vi "Wiener_HV_PowerSupplyWithLabVIEW.vi"() -> ()   [LabVIEW 2018]
panel:
  out "Numeric":i32
  in  "Tab Control":T1(tab)
  in  "IP":string="192.168.0.250"
  in  "stop":bool
  out "S1_Current":dbl[](array[numeric])
  out "S1_Voltage":dbl[](array[numeric])
  out "S2_Voltage":dbl[](array[numeric])
  out "S2_Current":dbl[](array[numeric])
  out "Start Time_L1":string
  out "S1_6-12 Channels Voltage":cluster{timestamp[], dbl[]}[](graph)
  out "S1_1-6 Channels Voltage":cluster{timestamp[], dbl[]}[](graph)
  out "S1_13-16 Channels Voltage":cluster{timestamp[], dbl[]}[](graph)
  in  "Clear_L1":bool
  out "Start Time_L2":string
  out "S1_13-16 Channels Current":cluster{timestamp[], dbl[]}[](graph)
  out "S1_1-6 Channels Current":cluster{timestamp[], dbl[]}[](graph)
  out "S1_6-12 Channels Current":cluster{timestamp[], dbl[]}[](graph)
  in  "Clear_L2":bool
  out "Start Time_L3":string
  out "S2_13-16 Channels Voltage":cluster{timestamp[], dbl[]}[](graph)
  out "S2_6-12 Channels Voltage":cluster{timestamp[], dbl[]}[](graph)
  out "S2_1-6 Channels Voltage":cluster{timestamp[], dbl[]}[](graph)
  in  "Clear_L3":bool
  out "Start Time_L4":string
  out "S2_1-6 Channels Current":cluster{timestamp[], dbl[]}[](graph)
  out "S2_6-12 Channels Current":cluster{timestamp[], dbl[]}[](graph)
  out "S2_13-16 Channels Current":cluster{timestamp[], dbl[]}[](graph)
  in  "Clear_L4":bool
  out "S1_V13":dbl format="%.2f"
  out "S1_V12":dbl format="%.2f"
  out "S1_V15":dbl format="%.2f"
  out "S1_V14":dbl format="%.2f"
  out "S1_I13":dbl format="%.2f"
  out "S1_I12":dbl format="%.2f"
  out "S1_I15":dbl format="%.2f"
  out "S1_I14":dbl format="%.2f"
  out "S1_I9":dbl format="%.2f"
  out "S1_I8":dbl format="%.2f"
  out "S1_I7":dbl format="%.2f"
  out "S1_I6":dbl format="%.2f"
  out "S1_V11":dbl format="%.2f"
  out "S1_V10":dbl format="%.2f"
  out "S1_V9":dbl format="%.2f"
  out "S1_V8":dbl format="%.2f"
  out "S1_V7":dbl format="%.2f"
  out "S1_V6":dbl format="%.2f"
  out "S1_I5":dbl format="%.2f"
  out "S1_I4":dbl format="%.2f"
  out "S1_I3":dbl format="%.2f"
  out "S1_I2":dbl format="%.2f"
  out "S1_I1":dbl format="%.2f"
  out "S1_V0":dbl format="%.2f"
  out "S1_V1":dbl format="%.2f"
  out "S1_V2":dbl format="%.2f"
  out "S1_V3":dbl format="%.2f"
  out "S1_V5":dbl format="%.2f"
  out "S1_V4":dbl format="%.2f"
  out "S1_I0":dbl format="%.2f"
  out "S1_I11":dbl format="%.2f"
  out "S1_I10":dbl format="%.2f"
  out "S2_V6":dbl format="%.2f"
  out "S2_V7":dbl format="%.2f"
  out "S2_V8":dbl format="%.2f"
  out "S2_V9":dbl format="%.2f"
  out "S2_V10":dbl format="%.2f"
  out "S2_V11":dbl format="%.2f"
  out "S2_I0":dbl format="%.2f"
  out "S2_I1":dbl format="%.2f"
  out "S2_I2":dbl format="%.2f"
  out "S2_I3":dbl format="%.2f"
  out "S2_I4":dbl format="%.2f"
  out "S2_I5":dbl format="%.2f"
  out "S2_I6":dbl format="%.2f"
  out "S2_I7":dbl format="%.2f"
  out "S2_I8":dbl format="%.2f"
  out "S2_I9":dbl format="%.2f"
  out "S2_I10":dbl format="%.2f"
  out "S2_I11":dbl format="%.2f"
  out "S2_I14":dbl format="%.2f"
  out "S2_I15":dbl format="%.2f"
  out "S2_I12":dbl format="%.2f"
  out "S2_I13":dbl format="%.2f"
  out "S2_V14":dbl format="%.2f"
  out "S2_V15":dbl format="%.2f"
  out "S2_V12":dbl format="%.2f"
  out "S2_V13":dbl format="%.2f"
  out "S2_V0":dbl format="%.2f"
  out "S2_V1":dbl format="%.2f"
  out "S2_V2":dbl format="%.2f"
  out "S2_V3":dbl format="%.2f"
  out "S2_V4":dbl format="%.2f"
  out "S2_V5":dbl format="%.2f"
  # "uA"
  # "V"
  # "uA"
  # "V"
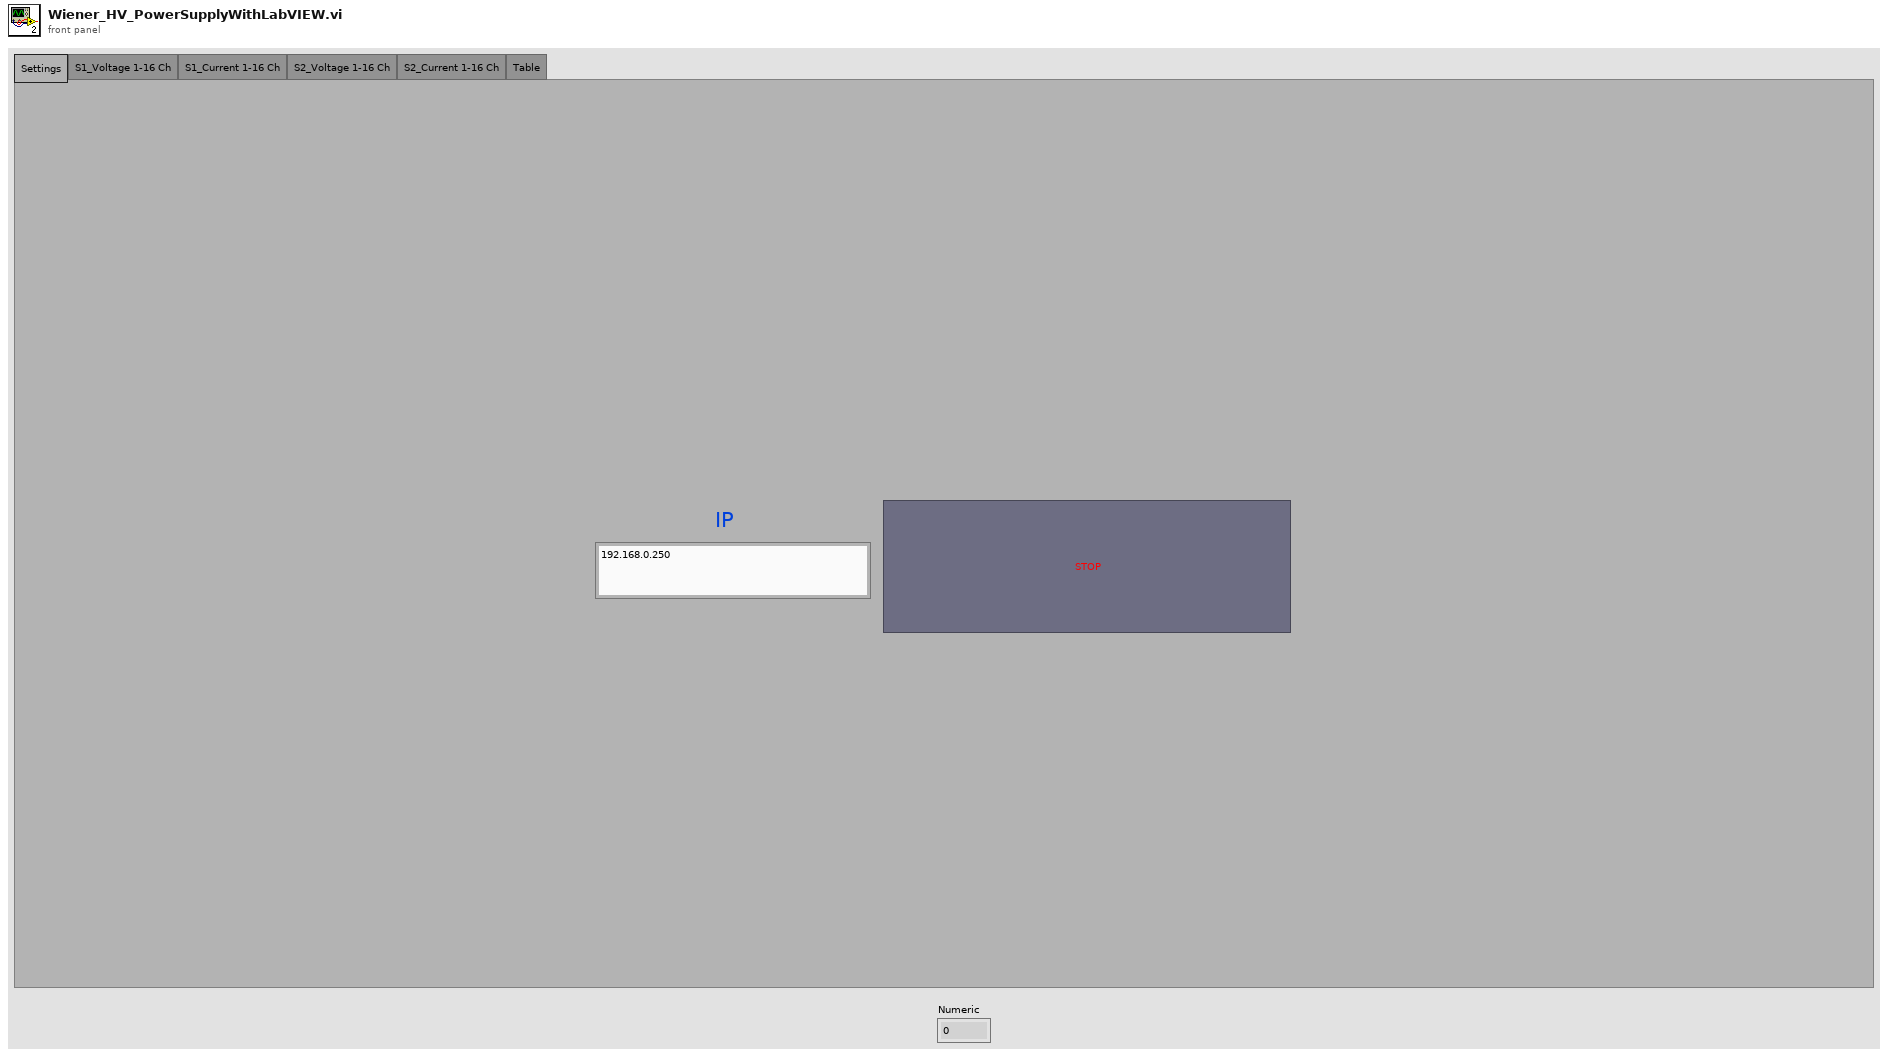
[diagram p1: front panel]
types:
  T1 = enum32{"Settings", "S1_Voltage 1-16 Ch", "S1_Current 1-16 Ch", "S2_Voltage 1-16 Ch", "S2_Current 1-16 Ch", "Table"}
  T2 = typedef "LVDateTimeRec.ctl" = cluster{"fractional second":dbl, "second":i32, "minute":i32, "hour":i32, "day of month":i32, "month":i32, "year":i32, "day of week":i32, "day of year":i32, "DST":i32}
  T3 = cluster{dbl, i32, i32, i32, "day of month":i32, "month":i32, "year":i32, "day of week":i32, "day of year":i32, "DST":i32}
  T4 = cluster{"fractional second":dbl, i32, i32, i32, "day of month":i32, "month":i32, "year":i32, "day of week":i32, "day of year":i32, "DST":i32}
  T5 = cluster{"appended array":timestamp[], "Ch 11":dbl[]}[]
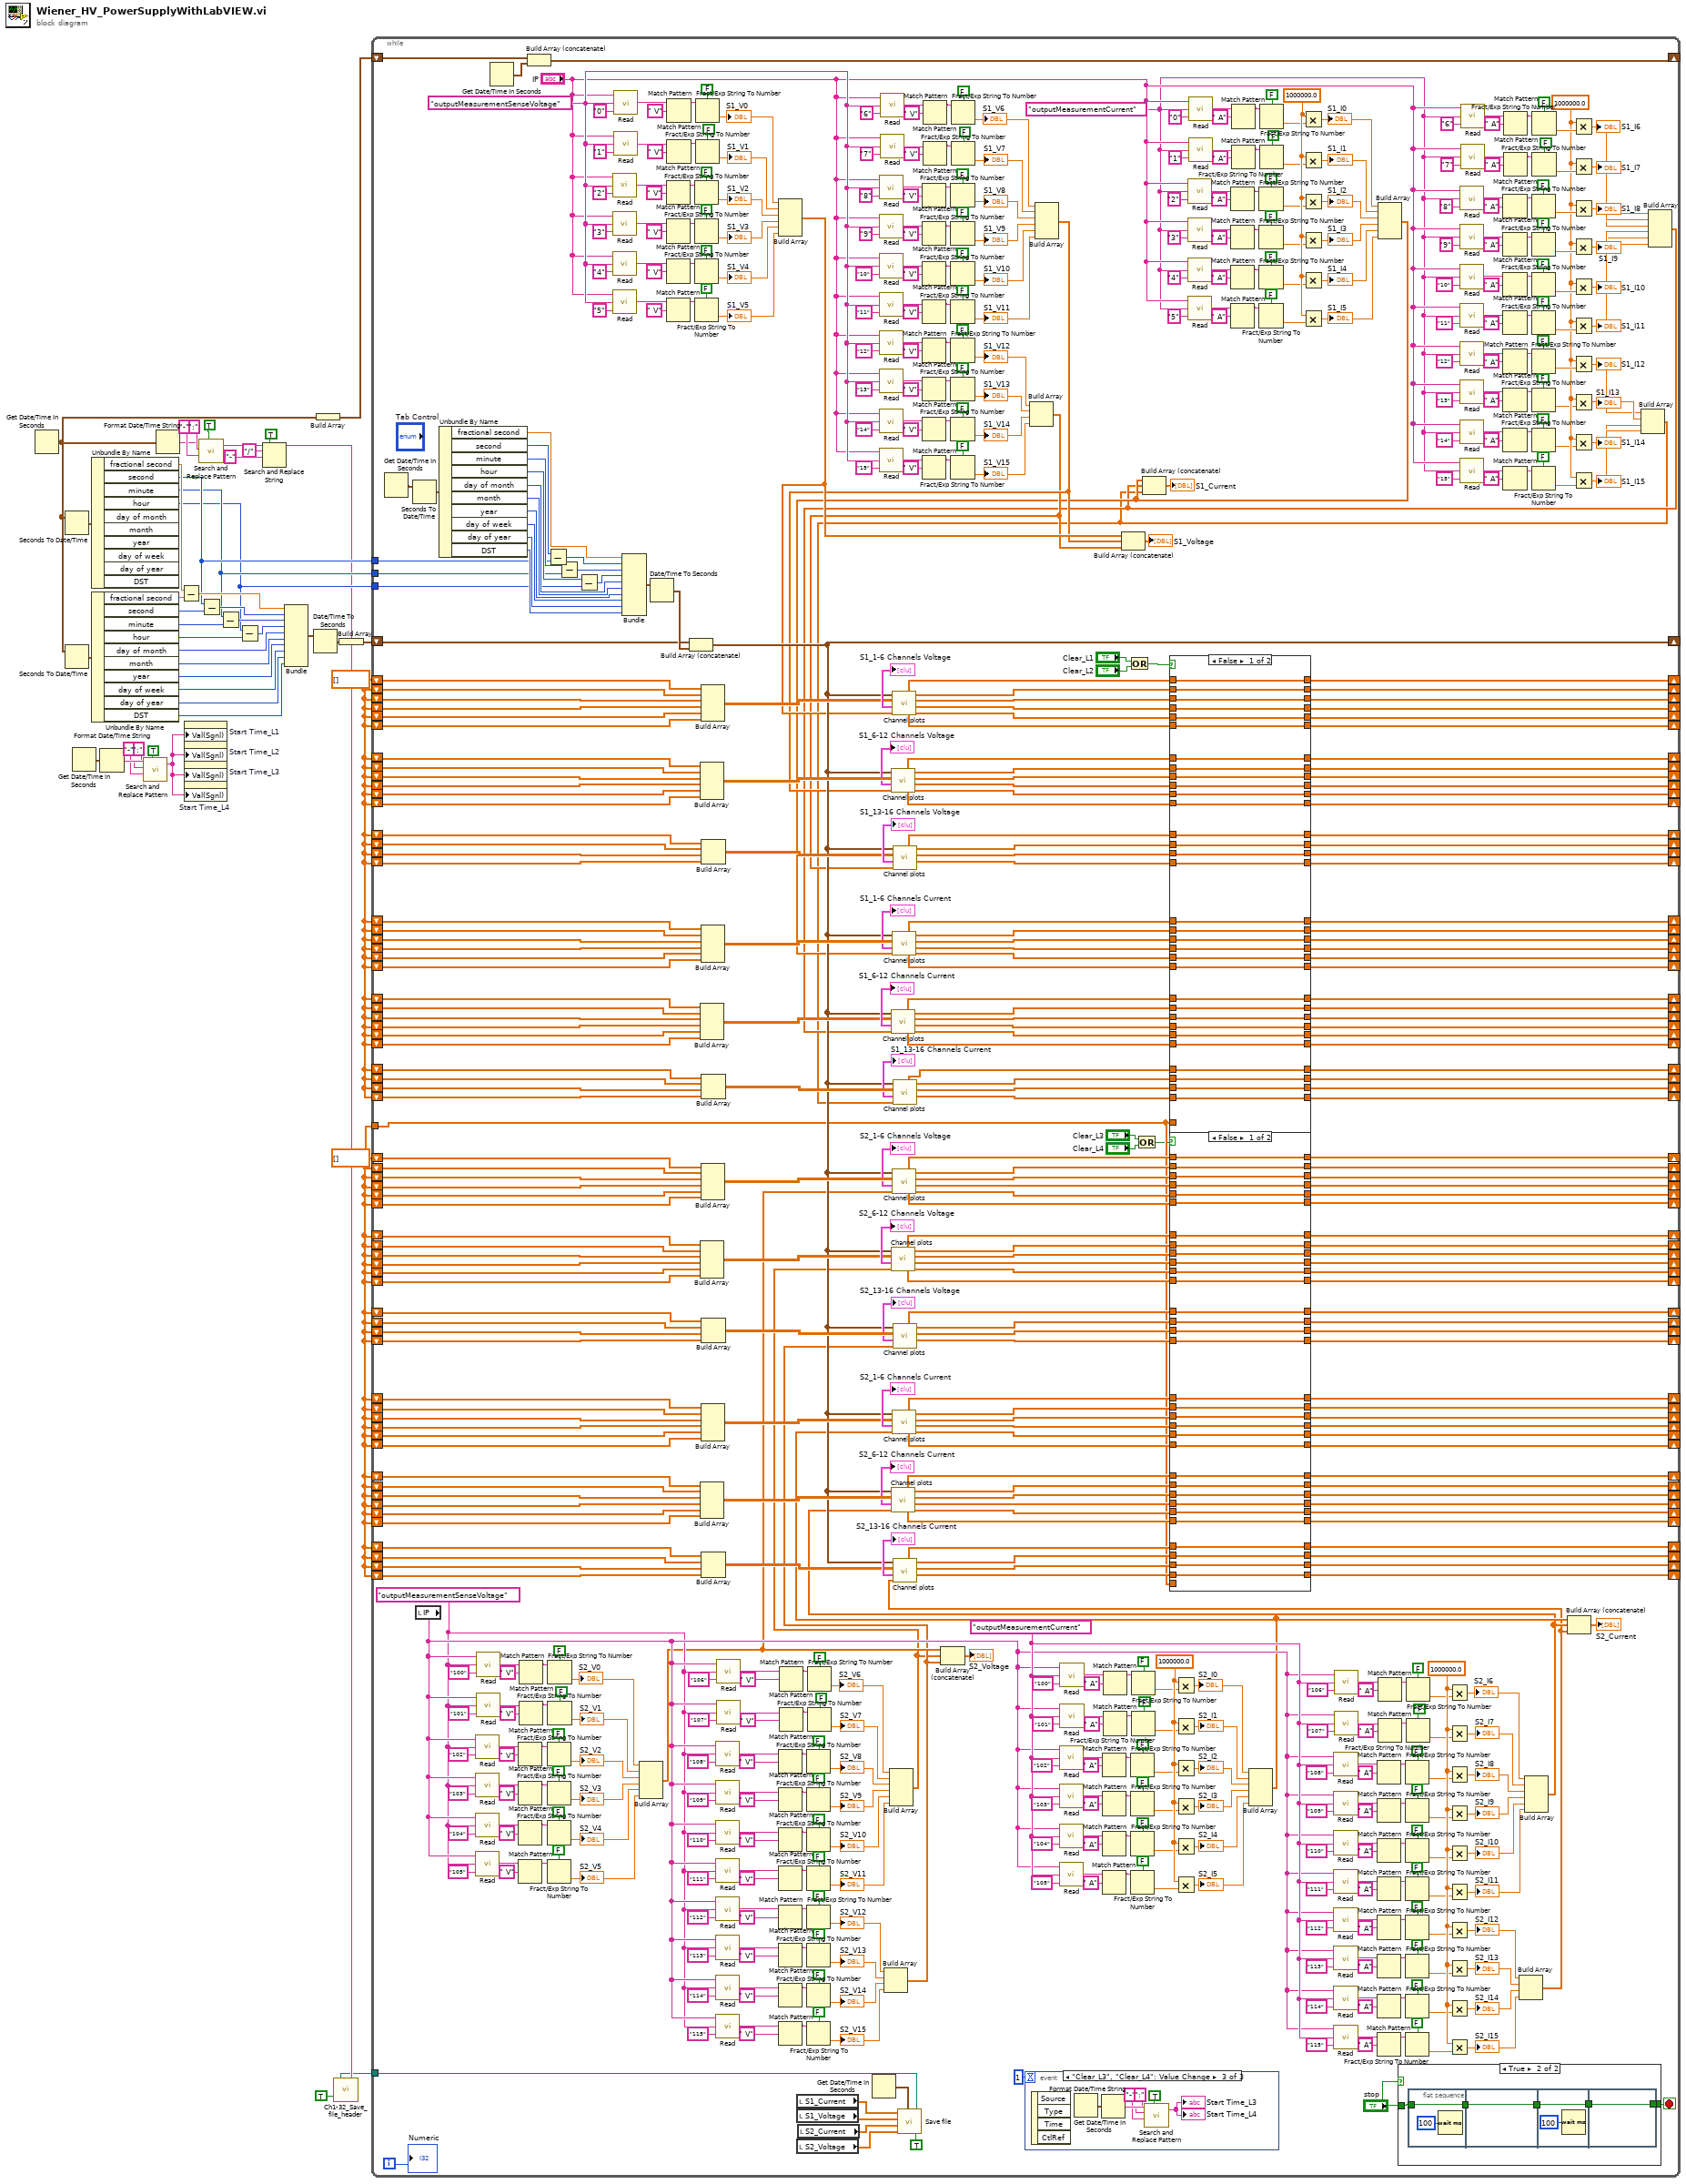
[diagram p0: block diagram]
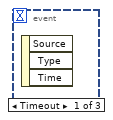
[diagram p3: hidden frame]
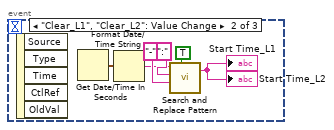
[diagram p4: hidden frame]
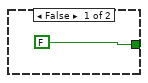
[diagram p6: hidden frame]
diagram:
  w8 = dbl[] [] ("out Ch 1")
  w15 = dbl[] [] ("out Ch 1")
  n1 = Get Date/Time In Seconds() -> (seconds since 1Jan1904=w18:timestamp)
  n2 = Seconds To Date/Time(time stamp (now)=w18) -> (date time rec=w26:T2)  [unwired: 1 in]
  n3 = Seconds To Date/Time(time stamp (now)=w18) -> (date time rec=w44:T2)  [unwired: 1 in]
  n4 = Get Date/Time In Seconds() -> (seconds since 1Jan1904=w6:timestamp)
  n5 = Unbundle By Name(w26) -> ("fractional second"=w29:dbl, "second"=w21:i32, "minute"=w20:i32, "hour"=w19:i32)  [unwired: 6 out]
  n6 = Unbundle By Name(w44) -> ("fractional second"=w43:dbl, "second"=w42:i32, "minute"=w41:i32, "hour"=w40:i32, "day of month"=w28:i32, "month"=w27:i32, "year"=w35:i32, "day of week"=w34:i32, "day of year"=w33:i32, "DST"=w32:i32)
  n7 = Format Date/Time String(seconds (now)=w6) -> (date/time string=w5:string)  [unwired: 2 in]
  n8 = call <vilib>:"Search and Replace Pattern.vi"("string"=w5, "regular expression (\"\")"=":" ("regular expression (\"\")"), "replace string (\"\")"="-" ("replace string (\"\")"), "replace all? (F)"=TRUE) -> ("result string"=w2:string)  [unwired: 1 in, 1 out]
  n9 = Format Date/Time String(seconds (now)=w18) -> (date/time string=w22:string)  [unwired: 2 in]
  n10 = Subtract(x=w29, y=w43) -> (x-y=w39:dbl)
  n11 = property on="Start Time_L1" class="Str"("Val(Sgnl)"=w2) -> ()  [unwired: 2 in, 2 out]
  n12 = property on="Start Time_L2" class="Str"("Val(Sgnl)"=w2) -> ()  [unwired: 2 in, 2 out]
  n13 = property on="Start Time_L3" class="Str"("Val(Sgnl)"=w2) -> ()  [unwired: 2 in, 2 out]
  n14 = property on="Start Time_L4" class="Str"("Val(Sgnl)"=w2) -> ()  [unwired: 2 in, 2 out]
  n15 = call <vilib>:"Search and Replace Pattern.vi"("string"=w22, "regular expression (\"\")"=":" ("regular expression (\"\")"), "replace string (\"\")"="-" ("replace string (\"\")"), "replace all? (F)"=TRUE) -> ("result string"=w13:string)  [unwired: 1 in, 1 out]
  n16 = Subtract(x=w21, y=w42) -> (x-y=w38:i32)
  n17 = Subtract(x=w20, y=w41) -> (x-y=w37:i32)
  n18 = Subtract(x=w19, y=w40) -> (x-y=w36:i32)
  n19 = Search and Replace String(replace all?=TRUE ("replace all? (F)"), input string=w13, search string="/", replace string="-" ("replace string (\"\")")) -> (result string=w9:string)  [unwired: 4 in, 3 out]
  n20 = Bundle(w39, w38, w37, w36, "day of month"=w28, "month"=w27, "year"=w35, "day of week"=w34, "day of year"=w33, "DST"=w32) -> (w30:T3)  [unwired: 1 in]
  n21 = Date/Time To Seconds(2:w30) -> (0:w31:timestamp)  [unwired: 1 in]
  n22 = Build Array(w18) -> (w17:timestamp[])
  n23 = call "Ch1-32_Save_file_header.vi"("File name"=w9, "Save"=TRUE) -> ("Output Path"=w1:path)
  n24 = Build Array(w31) -> (w16:timestamp[])
  n25 = while {
    tunnel: w21 -> [w725]
    tunnel: w20 -> [w724]
    tunnel: w19 -> [w723]
    shift-right: [w720] -> _
    shift-left: w17 -> [w722]
    shift-right: [w460] -> _
    shift-left: w16 -> [w718]
    shift-right: [w262] -> _
    shift-left: w15 -> [w715]
    shift-right: [w261] -> _
    shift-left: w15 -> [w714]
    shift-right: [w258] -> _
    shift-left: w15 -> [w713]
    shift-right: [w256] -> _
    shift-left: w15 -> [w712]
    shift-right: [w254] -> _
    shift-left: w15 -> [w711]
    shift-right: [w253] -> _
    shift-left: w15 -> [w710]
    shift-right: [w250] -> _
    shift-left: w15 -> [w642]
    shift-right: [w248] -> _
    shift-left: w15 -> [w643]
    shift-right: [w246] -> _
    shift-left: w15 -> [w644]
    shift-right: [w244] -> _
    shift-left: w15 -> [w645]
    shift-right: [w242] -> _
    shift-left: w15 -> [w646]
    shift-right: [w240] -> _
    shift-left: w15 -> [w647]
    shift-right: [w230] -> _
    shift-left: w15 -> [w566]
    shift-right: [w228] -> _
    shift-left: w15 -> [w567]
    shift-right: [w226] -> _
    shift-left: w15 -> [w568]
    shift-right: [w224] -> _
    shift-left: w15 -> [w569]
    shift-right: [w222] -> _
    shift-left: w15 -> [w570]
    shift-right: [w220] -> _
    shift-left: w15 -> [w571]
    shift-right: [w218] -> _
    shift-left: w15 -> [w577]
    shift-right: [w216] -> _
    shift-left: w15 -> [w576]
    shift-right: [w214] -> _
    shift-left: w15 -> [w575]
    shift-right: [w212] -> _
    shift-left: w15 -> [w574]
    shift-right: [w210] -> _
    shift-left: w15 -> [w573]
    shift-right: [w208] -> _
    shift-left: w15 -> [w572]
    shift-right: [w238] -> _
    shift-left: w15 -> [w561]
    shift-right: [w236] -> _
    shift-left: w15 -> [w560]
    shift-right: [w234] -> _
    shift-left: w15 -> [w559]
    shift-right: [w232] -> _
    shift-left: w15 -> [w558]
    shift-right: [w206] -> _
    shift-left: w15 -> [w507]
    shift-right: [w204] -> _
    shift-left: w15 -> [w508]
    shift-right: [w202] -> _
    shift-left: w15 -> [w509]
    shift-right: [w200] -> _
    shift-left: w15 -> [w510]
    shift-right: [w194] -> _
    shift-left: w8 -> [w463]
    shift-right: [w192] -> _
    shift-left: w8 -> [w464]
    shift-right: [w190] -> _
    shift-left: w8 -> [w465]
    shift-right: [w188] -> _
    shift-left: w8 -> [w466]
    shift-right: [w186] -> _
    shift-left: w8 -> [w467]
    shift-right: [w184] -> _
    shift-left: w8 -> [w468]
    shift-right: [w182] -> _
    shift-left: w8 -> [w474]
    shift-right: [w180] -> _
    shift-left: w8 -> [w473]
    shift-right: [w178] -> _
    shift-left: w8 -> [w472]
    shift-right: [w176] -> _
    shift-left: w8 -> [w471]
    shift-right: [w174] -> _
    shift-left: w8 -> [w470]
    shift-right: [w172] -> _
    shift-left: w8 -> [w469]
    shift-right: [w162] -> _
    shift-left: w8 -> [w490]
    shift-right: [w160] -> _
    shift-left: w8 -> [w489]
    shift-right: [w158] -> _
    shift-left: w8 -> [w488]
    shift-right: [w156] -> _
    shift-left: w8 -> [w487]
    shift-right: [w154] -> _
    shift-left: w8 -> [w486]
    shift-right: [w152] -> _
    shift-left: w8 -> [w485]
    shift-right: [w150] -> _
    shift-left: w8 -> [w479]
    shift-right: [w148] -> _
    shift-left: w8 -> [w480]
    shift-right: [w146] -> _
    shift-left: w8 -> [w481]
    shift-right: [w144] -> _
    shift-left: w8 -> [w482]
    shift-right: [w142] -> _
    shift-left: w8 -> [w483]
    shift-right: [w140] -> _
    shift-left: w8 -> [w484]
    shift-right: [w170] -> _
    shift-left: w8 -> [w495]
    shift-right: [w168] -> _
    shift-left: w8 -> [w496]
    shift-right: [w166] -> _
    shift-left: w8 -> [w497]
    shift-right: [w164] -> _
    shift-left: w8 -> [w498]
    shift-right: [w138] -> _
    shift-left: w8 -> [w502]
    shift-right: [w136] -> _
    shift-left: w8 -> [w501]
    shift-right: [w134] -> _
    shift-left: w8 -> [w500]
    shift-right: [w132] -> _
    shift-left: w8 -> [w499]
    tunnel: w8 -> [w130]
    tunnel: w1 -> [w47]
    i -> [w45]
    stop <- w264 stop-if-true
    w73 = 1000000.0 ("x")
    w86 = 1000000.0 ("x")
    w93 = 1000000.0 ("x")
    w126 = 1000000.0 ("x")
    w281 = "outputMeasurementSenseVoltage" ("R_Call_Function_Voltage")
    w283 = "outputMeasurementCurrent" ("R_Call_Function_Voltage")
    w511 = "outputMeasurementCurrent" ("R_Call_Function_Voltage")
    w537 = "outputMeasurementSenseVoltage" ("R_Call_Function_Voltage")
    n26 = Get Date/Time In Seconds() -> (seconds since 1Jan1904=w741:timestamp)
    n27 = Seconds To Date/Time(time stamp (now)=w741) -> (date time rec=w740:T2)  [unwired: 1 in]
    n28 = local read "IP"() -> (w282:string)
    n29 = Unbundle By Name(w740) -> ("fractional second"=w726:dbl, "second"=w736:i32, "minute"=w735:i32, "hour"=w734:i32, "day of month"=w733:i32, "month"=w732:i32, "year"=w731:i32, "day of week"=w730:i32, "day of year"=w729:i32, "DST"=w728:i32)
    n30 = call "Read.vi"("R_Channel"="102", "R_Call_Function"=w281, "IP"=w282) -> ("R_Return"=w447:string)
    n31 = call "Read.vi"("R_Channel"="103", "R_Call_Function"=w281, "IP"=w282) -> ("R_Return"=w445:string)
    n32 = call "Read.vi"("R_Channel"="104", "R_Call_Function"=w281, "IP"=w282) -> ("R_Return"=w435:string)
    n33 = call "Read.vi"("R_Channel"="105", "R_Call_Function"=w281, "IP"=w282) -> ("R_Return"=w436:string)
    n34 = call "Read.vi"("R_Channel"="100", "R_Call_Function"=w281, "IP"=w282) -> ("R_Return"=w456:string)
    n35 = call "Read.vi"("R_Channel"="101", "R_Call_Function"=w281, "IP"=w282) -> ("R_Return"=w446:string)
    n36 = Get Date/Time In Seconds() -> (seconds since 1Jan1904=w721:timestamp)
    n37 = Match Pattern(string=w447, regular expression=" V") -> (before substring=w448:string)  [unwired: 1 in, 3 out]
    n38 = Match Pattern(string=w445, regular expression=" V") -> (before substring=w444:string)  [unwired: 1 in, 3 out]
    n39 = Match Pattern(string=w435, regular expression=" V") -> (before substring=w434:string)  [unwired: 1 in, 3 out]
    n40 = Match Pattern(string=w436, regular expression=" V") -> (before substring=w437:string)  [unwired: 1 in, 3 out]
    n41 = Match Pattern(string=w456, regular expression=" V") -> (before substring=w457:string)  [unwired: 1 in, 3 out]
    n42 = Match Pattern(string=w446, regular expression=" V") -> (before substring=w455:string)  [unwired: 1 in, 3 out]
    n43 = Build Array (concatenate)(w722, w721) -> (w720:timestamp[])
    n44 = Subtract(x=w736, y=w725) -> (x-y=w737:i32)
    n45 = Fract/Exp String To Number(use system decimal point (T)=FALSE, string=w448) -> (number=w428:dbl)  [unwired: 2 in, 1 out]
    "S2_V2" <- w428
    n46 = Fract/Exp String To Number(use system decimal point (T)=FALSE, string=w444) -> (number=w427:dbl)  [unwired: 2 in, 1 out]
    "S2_V3" <- w427
    n47 = Fract/Exp String To Number(use system decimal point (T)=FALSE, string=w434) -> (number=w426:dbl)  [unwired: 2 in, 1 out]
    "S2_V4" <- w426
    n48 = Fract/Exp String To Number(use system decimal point (T)=FALSE, string=w437) -> (number=w425:dbl)  [unwired: 2 in, 1 out]
    "S2_V5" <- w425
    n49 = Fract/Exp String To Number(use system decimal point (T)=FALSE, string=w457) -> (number=w430:dbl)  [unwired: 2 in, 1 out]
    "S2_V0" <- w430
    n50 = Fract/Exp String To Number(use system decimal point (T)=FALSE, string=w455) -> (number=w429:dbl)  [unwired: 2 in, 1 out]
    "S2_V1" <- w429
    n51 = Subtract(x=w735, y=w724) -> (x-y=w738:i32)
    n52 = Subtract(x=w734, y=w723) -> (x-y=w739:i32)
    n53 = call "Read.vi"("R_Channel"="2", "R_Call_Function"=w537, "IP"="IP") -> ("R_Return"=w701:string)
    n54 = call "Read.vi"("R_Channel"="3", "R_Call_Function"=w537, "IP"="IP") -> ("R_Return"=w699:string)
    n55 = call "Read.vi"("R_Channel"="4", "R_Call_Function"=w537, "IP"="IP") -> ("R_Return"=w689:string)
    n56 = call "Read.vi"("R_Channel"="5", "R_Call_Function"=w537, "IP"="IP") -> ("R_Return"=w690:string)
    n57 = call "Read.vi"("R_Channel"="0", "R_Call_Function"=w537, "IP"="IP") -> ("R_Return"=w742:string)
    n58 = call "Read.vi"("R_Channel"="1", "R_Call_Function"=w537, "IP"="IP") -> ("R_Return"=w700:string)
    n59 = Bundle("fractional second"=w726, w737, w738, w739, "day of month"=w733, "month"=w732, "year"=w731, "day of week"=w730, "day of year"=w729, "DST"=w728) -> (w727:T4)  [unwired: 1 in]
    n60 = Build Array(w430, w429, w428, w427, w426, w425) -> (w274:dbl[])
    n61 = Date/Time To Seconds(2:w727) -> (0:w719:timestamp)  [unwired: 1 in]
    n62 = Match Pattern(string=w701, regular expression=" V") -> (before substring=w702:string)  [unwired: 1 in, 3 out]
    n63 = Match Pattern(string=w699, regular expression=" V") -> (before substring=w698:string)  [unwired: 1 in, 3 out]
    n64 = Match Pattern(string=w689, regular expression=" V") -> (before substring=w688:string)  [unwired: 1 in, 3 out]
    n65 = Match Pattern(string=w690, regular expression=" V") -> (before substring=w691:string)  [unwired: 1 in, 3 out]
    n66 = Match Pattern(string=w742, regular expression=" V") -> (before substring=w743:string)  [unwired: 1 in, 3 out]
    n67 = Match Pattern(string=w700, regular expression=" V") -> (before substring=w709:string)  [unwired: 1 in, 3 out]
    n68 = Build Array (concatenate)(w718, w719) -> (w460:timestamp[])
    n69 = Fract/Exp String To Number(use system decimal point (T)=FALSE, string=w702) -> (number=w122:dbl)  [unwired: 2 in, 1 out]
    "S1_V2" <- w122
    n70 = Fract/Exp String To Number(use system decimal point (T)=FALSE, string=w698) -> (number=w123:dbl)  [unwired: 2 in, 1 out]
    "S1_V3" <- w123
    n71 = Fract/Exp String To Number(use system decimal point (T)=FALSE, string=w688) -> (number=w125:dbl)  [unwired: 2 in, 1 out]
    "S1_V4" <- w125
    n72 = Fract/Exp String To Number(use system decimal point (T)=FALSE, string=w691) -> (number=w124:dbl)  [unwired: 2 in, 1 out]
    "S1_V5" <- w124
    n73 = Fract/Exp String To Number(use system decimal point (T)=FALSE, string=w743) -> (number=w120:dbl)  [unwired: 2 in, 1 out]
    "S1_V0" <- w120
    n74 = Fract/Exp String To Number(use system decimal point (T)=FALSE, string=w709) -> (number=w121:dbl)  [unwired: 2 in, 1 out]
    "S1_V1" <- w121
    n75 = Build Array(w642, w643, w644, w645, w646, w647) -> (w641:dbl[][])
    n76 = Build Array(w577, w576, w575, w574, w573, w572) -> (w578:dbl[][])
    n77 = Build Array(w474, w473, w472, w471, w470, w469) -> (w475:dbl[][])
    n78 = Build Array(w479, w480, w481, w482, w483, w484) -> (w478:dbl[][])
    n79 = Build Array(w715, w714, w713, w712, w711, w710) -> (w716:dbl[][])
    n80 = Build Array(w566, w567, w568, w569, w570, w571) -> (w565:dbl[][])
    n81 = Build Array(w463, w464, w465, w466, w467, w468) -> (w462:dbl[][])
    n82 = Build Array(w490, w489, w488, w487, w486, w485) -> (w491:dbl[][])
    n83 = Build Array(w561, w560, w559, w558) -> (w562:dbl[][])
    n84 = Build Array(w507, w508, w509, w510) -> (w506:dbl[][])
    n85 = Build Array(w495, w496, w497, w498) -> (w494:dbl[][])
    n86 = Build Array(w502, w501, w500, w499) -> (w503:dbl[][])
    n87 = call "Read.vi"("R_Channel"="108", "R_Call_Function"=w281, "IP"=w282) -> ("R_Return"=w400:string)
    n88 = call "Read.vi"("R_Channel"="109", "R_Call_Function"=w281, "IP"=w282) -> ("R_Return"=w402:string)
    n89 = call "Read.vi"("R_Channel"="110", "R_Call_Function"=w281, "IP"=w282) -> ("R_Return"=w412:string)
    n90 = call "Read.vi"("R_Channel"="111", "R_Call_Function"=w281, "IP"=w282) -> ("R_Return"=w411:string)
    n91 = call "Read.vi"("R_Channel"="112", "R_Call_Function"=w281, "IP"=w282) -> ("R_Return"=w323:string)
    n92 = call "Read.vi"("R_Channel"="113", "R_Call_Function"=w281, "IP"=w282) -> ("R_Return"=w322:string)
    n93 = call "Read.vi"("R_Channel"="114", "R_Call_Function"=w281, "IP"=w282) -> ("R_Return"=w312:string)
    n94 = call "Read.vi"("R_Channel"="115", "R_Call_Function"=w281, "IP"=w282) -> ("R_Return"=w313:string)
    n95 = call "Read.vi"("R_Channel"="106", "R_Call_Function"=w281, "IP"=w282) -> ("R_Return"=w391:string)
    n96 = call "Read.vi"("R_Channel"="107", "R_Call_Function"=w281, "IP"=w282) -> ("R_Return"=w401:string)
    n97 = Build Array(w120, w121, w122, w123, w125, w124) -> (w280:dbl[])
    n98 = Match Pattern(string=w400, regular expression=" V") -> (before substring=w399:string)  [unwired: 1 in, 3 out]
    n99 = Match Pattern(string=w402, regular expression=" V") -> (before substring=w403:string)  [unwired: 1 in, 3 out]
    n100 = Match Pattern(string=w412, regular expression=" V") -> (before substring=w413:string)  [unwired: 1 in, 3 out]
    n101 = Match Pattern(string=w411, regular expression=" V") -> (before substring=w410:string)  [unwired: 1 in, 3 out]
    n102 = Match Pattern(string=w323, regular expression=" V") -> (before substring=w324:string)  [unwired: 1 in, 3 out]
    n103 = Match Pattern(string=w322, regular expression=" V") -> (before substring=w321:string)  [unwired: 1 in, 3 out]
    n104 = Match Pattern(string=w312, regular expression=" V") -> (before substring=w311:string)  [unwired: 1 in, 3 out]
    n105 = Match Pattern(string=w313, regular expression=" V") -> (before substring=w314:string)  [unwired: 1 in, 3 out]
    n106 = Match Pattern(string=w391, regular expression=" V") -> (before substring=w390:string)  [unwired: 1 in, 3 out]
    n107 = Match Pattern(string=w401, regular expression=" V") -> (before substring=w392:string)  [unwired: 1 in, 3 out]
    n108 = local read "S1_Current"() -> (w49:dbl[])
    n109 = local read "S1_Voltage"() -> (w50:dbl[])
    n110 = local read "S2_Voltage"() -> (w52:dbl[])
    n111 = local read "S2_Current"() -> (w51:dbl[])
    n112 = Fract/Exp String To Number(use system decimal point (T)=FALSE, string=w399) -> (number=w419:dbl)  [unwired: 2 in, 1 out]
    "S2_V8" <- w419
    n113 = Fract/Exp String To Number(use system decimal point (T)=FALSE, string=w403) -> (number=w420:dbl)  [unwired: 2 in, 1 out]
    "S2_V9" <- w420
    n114 = Fract/Exp String To Number(use system decimal point (T)=FALSE, string=w413) -> (number=w421:dbl)  [unwired: 2 in, 1 out]
    "S2_V10" <- w421
    n115 = Fract/Exp String To Number(use system decimal point (T)=FALSE, string=w410) -> (number=w422:dbl)  [unwired: 2 in, 1 out]
    "S2_V11" <- w422
    n116 = Fract/Exp String To Number(use system decimal point (T)=FALSE, string=w324) -> (number=w307:dbl)  [unwired: 2 in, 1 out]
    "S2_V12" <- w307
    n117 = Fract/Exp String To Number(use system decimal point (T)=FALSE, string=w321) -> (number=w306:dbl)  [unwired: 2 in, 1 out]
    "S2_V13" <- w306
    n118 = Fract/Exp String To Number(use system decimal point (T)=FALSE, string=w311) -> (number=w305:dbl)  [unwired: 2 in, 1 out]
    "S2_V14" <- w305
    n119 = Fract/Exp String To Number(use system decimal point (T)=FALSE, string=w314) -> (number=w304:dbl)  [unwired: 2 in, 1 out]
    "S2_V15" <- w304
    n120 = Fract/Exp String To Number(use system decimal point (T)=FALSE, string=w390) -> (number=w417:dbl)  [unwired: 2 in, 1 out]
    "S2_V6" <- w417
    n121 = Fract/Exp String To Number(use system decimal point (T)=FALSE, string=w392) -> (number=w418:dbl)  [unwired: 2 in, 1 out]
    "S2_V7" <- w418
    n122 = Get Date/Time In Seconds() -> (seconds since 1Jan1904=w48:timestamp)
    n123 = call "Read.vi"("R_Channel"="8", "R_Call_Function"=w537, "IP"="IP") -> ("R_Return"=w660:string)
    n124 = call "Read.vi"("R_Channel"="9", "R_Call_Function"=w537, "IP"="IP") -> ("R_Return"=w662:string)
    n125 = call "Read.vi"("R_Channel"="10", "R_Call_Function"=w537, "IP"="IP") -> ("R_Return"=w672:string)
    n126 = call "Read.vi"("R_Channel"="11", "R_Call_Function"=w537, "IP"="IP") -> ("R_Return"=w671:string)
    n127 = call "Read.vi"("R_Channel"="12", "R_Call_Function"=w537, "IP"="IP") -> ("R_Return"=w553:string)
    n128 = call "Read.vi"("R_Channel"="13", "R_Call_Function"=w537, "IP"="IP") -> ("R_Return"=w552:string)
    n129 = call "Read.vi"("R_Channel"="14", "R_Call_Function"=w537, "IP"="IP") -> ("R_Return"=w542:string)
    n130 = call "Read.vi"("R_Channel"="15", "R_Call_Function"=w537, "IP"="IP") -> ("R_Return"=w543:string)
    n131 = call "Read.vi"("R_Channel"="6", "R_Call_Function"=w537, "IP"="IP") -> ("R_Return"=w651:string)
    n132 = call "Read.vi"("R_Channel"="7", "R_Call_Function"=w537, "IP"="IP") -> ("R_Return"=w661:string)
    n133 = Build Array(w307, w306, w305, w304) -> (w273:dbl[])
    n134 = Build Array(w417, w418, w419, w420, w421, w422) -> (w131:dbl[])
    n135 = call "Channel plots.vi"("Current time"=w460, "In Channels"=w475, "Input Channels"=w131) -> ("output graph"=→"S2_6-12 Channels Voltage":T5, "out Ch 1"=w183:dbl[], "out Ch 6"=w173:dbl[], "out Ch 2"=w181:dbl[], "out Ch 3"=w179:dbl[], "out Ch 4"=w177:dbl[], "out Ch 5"=w175:dbl[])
    n136 = call "Channel plots.vi"("Current time"=w460, "In Channels"=w716, "Input Channels"=w280) -> ("output graph"=→"S1_1-6 Channels Voltage":T5, "out Ch 1"=w263:dbl[], "out Ch 6"=w252:dbl[], "out Ch 2"=w260:dbl[], "out Ch 3"=w259:dbl[], "out Ch 4"=w257:dbl[], "out Ch 5"=w255:dbl[])
    n137 = call "Channel plots.vi"("Current time"=w460, "In Channels"=w462, "Input Channels"=w274) -> ("output graph"=→"S2_1-6 Channels Voltage":T5, "out Ch 1"=w195:dbl[], "out Ch 6"=w185:dbl[], "out Ch 2"=w193:dbl[], "out Ch 3"=w191:dbl[], "out Ch 4"=w189:dbl[], "out Ch 5"=w187:dbl[])
    n138 = call "Channel plots.vi"("Current time"=w460, "In Channels"=w494, "Input Channels"=w273) -> ("output graph"=→"S2_13-16 Channels Voltage":T5, "out Ch 1"=w171:dbl[], "out Ch 2"=w169:dbl[], "out Ch 3"=w167:dbl[], "out Ch 4"=w165:dbl[])  [unwired: 2 out]
    n139 = call "Save file.vi"("S1_Current"=w49, "S1_Voltage"=w50, "S2_Current"=w51, "S2_Voltage"=w52, "current time"=w48, "Save path"=w47, "Save"=TRUE) -> ()
    n140 = Match Pattern(string=w660, regular expression=" V") -> (before substring=w659:string)  [unwired: 1 in, 3 out]
    n141 = Match Pattern(string=w662, regular expression=" V") -> (before substring=w663:string)  [unwired: 1 in, 3 out]
    n142 = Match Pattern(string=w672, regular expression=" V") -> (before substring=w673:string)  [unwired: 1 in, 3 out]
    n143 = Match Pattern(string=w671, regular expression=" V") -> (before substring=w670:string)  [unwired: 1 in, 3 out]
    n144 = Match Pattern(string=w553, regular expression=" V") -> (before substring=w554:string)  [unwired: 1 in, 3 out]
    n145 = Match Pattern(string=w552, regular expression=" V") -> (before substring=w551:string)  [unwired: 1 in, 3 out]
    n146 = Match Pattern(string=w542, regular expression=" V") -> (before substring=w541:string)  [unwired: 1 in, 3 out]
    n147 = Match Pattern(string=w543, regular expression=" V") -> (before substring=w544:string)  [unwired: 1 in, 3 out]
    n148 = Match Pattern(string=w651, regular expression=" V") -> (before substring=w650:string)  [unwired: 1 in, 3 out]
    n149 = Match Pattern(string=w661, regular expression=" V") -> (before substring=w652:string)  [unwired: 1 in, 3 out]
    n150 = Build Array (concatenate)(w274, w131, w273) -> (→"S2_Voltage":dbl[])
    n151 = Fract/Exp String To Number(use system decimal point (T)=FALSE, string=w659) -> (number=w679:dbl)  [unwired: 2 in, 1 out]
    "S1_V8" <- w679
    n152 = Fract/Exp String To Number(use system decimal point (T)=FALSE, string=w663) -> (number=w680:dbl)  [unwired: 2 in, 1 out]
    "S1_V9" <- w680
    n153 = Fract/Exp String To Number(use system decimal point (T)=FALSE, string=w673) -> (number=w681:dbl)  [unwired: 2 in, 1 out]
    "S1_V10" <- w681
    n154 = Fract/Exp String To Number(use system decimal point (T)=FALSE, string=w670) -> (number=w682:dbl)  [unwired: 2 in, 1 out]
    "S1_V11" <- w682
    n155 = Fract/Exp String To Number(use system decimal point (T)=FALSE, string=w554) -> (number=w536:dbl)  [unwired: 2 in, 1 out]
    "S1_V12" <- w536
    n156 = Fract/Exp String To Number(use system decimal point (T)=FALSE, string=w551) -> (number=w535:dbl)  [unwired: 2 in, 1 out]
    "S1_V13" <- w535
    n157 = Fract/Exp String To Number(use system decimal point (T)=FALSE, string=w541) -> (number=w534:dbl)  [unwired: 2 in, 1 out]
    "S1_V14" <- w534
    n158 = Fract/Exp String To Number(use system decimal point (T)=FALSE, string=w544) -> (number=w533:dbl)  [unwired: 2 in, 1 out]
    "S1_V15" <- w533
    n159 = Fract/Exp String To Number(use system decimal point (T)=FALSE, string=w650) -> (number=w677:dbl)  [unwired: 2 in, 1 out]
    "S1_V6" <- w677
    n160 = Fract/Exp String To Number(use system decimal point (T)=FALSE, string=w652) -> (number=w678:dbl)  [unwired: 2 in, 1 out]
    "S1_V7" <- w678
    n161 = event shown="[2] \"Clear_L3\", \"Clear_L4\": Value Change" {
      selector: _ -> [_ _ _]
      dyn-events: _ -> [_ _ _]
      timeout: 1 -> [_ _ _]
      event Timeout {
        n162 = event-data() -> ()  [unwired: 1 in, 3 out]
      }
      event "Clear_L1", "Clear_L2": Value Change {
        n163 = event-data() -> ()  [unwired: 1 in, 5 out]
        n164 = Get Date/Time In Seconds() -> (seconds since 1Jan1904=w781:timestamp)
        n165 = Format Date/Time String(seconds (now)=w781) -> (date/time string=w782:string)  [unwired: 2 in]
        n166 = call <vilib>:"Search and Replace Pattern.vi"("string"=w782, "regular expression (\"\")"=":" ("regular expression (\"\")"), "replace string (\"\")"="-" ("replace string (\"\")"), "replace all? (F)"=TRUE) -> ("result string"=→"Start Time_L1" →"Start Time_L2":string)  [unwired: 1 in, 1 out]
      }
      event "Clear_L3", "Clear_L4": Value Change {
        n167 = event-data() -> ()  [unwired: 1 in, 4 out]
        n168 = Get Date/Time In Seconds() -> (seconds since 1Jan1904=w789:timestamp)
        n169 = Format Date/Time String(seconds (now)=w789) -> (date/time string=w790:string)  [unwired: 2 in]
        n170 = call <vilib>:"Search and Replace Pattern.vi"("string"=w790, "regular expression (\"\")"=":" ("regular expression (\"\")"), "replace string (\"\")"="-" ("replace string (\"\")"), "replace all? (F)"=TRUE) -> ("result string"=→"Start Time_L3" →"Start Time_L4":string)  [unwired: 1 in, 1 out]
      }
    }
    n171 = Build Array(w536, w535, w534, w533) -> (w278:dbl[])
    n172 = call "Channel plots.vi"("Current time"=w460, "In Channels"=w562, "Input Channels"=w278) -> ("output graph"=→"S1_13-16 Channels Voltage":T5, "out Ch 1"=w239:dbl[], "out Ch 2"=w237:dbl[], "out Ch 3"=w235:dbl[], "out Ch 4"=w233:dbl[])  [unwired: 2 out]
    n173 = Build Array(w677, w678, w679, w680, w681, w682) -> (w279:dbl[])
    n174 = call "Channel plots.vi"("Current time"=w460, "In Channels"=w641, "Input Channels"=w279) -> ("output graph"=→"S1_6-12 Channels Voltage":T5, "out Ch 1"=w251:dbl[], "out Ch 6"=w241:dbl[], "out Ch 2"=w249:dbl[], "out Ch 3"=w247:dbl[], "out Ch 4"=w245:dbl[], "out Ch 5"=w243:dbl[])
    n175 = call "Read.vi"("R_Channel"="102", "R_Call_Function"=w283, "IP"=w282) -> ("R_Return"=w340:string)
    n176 = call "Read.vi"("R_Channel"="103", "R_Call_Function"=w283, "IP"=w282) -> ("R_Return"=w342:string)
    n177 = call "Read.vi"("R_Channel"="104", "R_Call_Function"=w283, "IP"=w282) -> ("R_Return"=w352:string)
    n178 = call "Read.vi"("R_Channel"="105", "R_Call_Function"=w283, "IP"=w282) -> ("R_Return"=w351:string)
    n179 = call "Read.vi"("R_Channel"="100", "R_Call_Function"=w283, "IP"=w282) -> ("R_Return"=w331:string)
    n180 = call "Read.vi"("R_Channel"="101", "R_Call_Function"=w283, "IP"=w282) -> ("R_Return"=w341:string)
    n181 = Match Pattern(string=w340, regular expression=" A") -> (before substring=w339:string)  [unwired: 1 in, 3 out]
    n182 = Match Pattern(string=w342, regular expression=" A") -> (before substring=w343:string)  [unwired: 1 in, 3 out]
    n183 = Match Pattern(string=w352, regular expression=" A") -> (before substring=w353:string)  [unwired: 1 in, 3 out]
    n184 = Match Pattern(string=w351, regular expression=" A") -> (before substring=w350:string)  [unwired: 1 in, 3 out]
    n185 = Match Pattern(string=w331, regular expression=" A") -> (before substring=w330:string)  [unwired: 1 in, 3 out]
    n186 = Match Pattern(string=w341, regular expression=" A") -> (before substring=w332:string)  [unwired: 1 in, 3 out]
    n187 = Build Array (concatenate)(w280, w279, w278) -> (→"S1_Voltage":dbl[])
    n188 = Or(x="Clear_L1", y="Clear_L2") -> (x .or. y?=w197:bool)
    n189 = Fract/Exp String To Number(use system decimal point (T)=FALSE, string=w339) -> (number=w78:dbl)  [unwired: 2 in, 1 out]
    n190 = Fract/Exp String To Number(use system decimal point (T)=FALSE, string=w343) -> (number=w76:dbl)  [unwired: 2 in, 1 out]
    n191 = Fract/Exp String To Number(use system decimal point (T)=FALSE, string=w353) -> (number=w83:dbl)  [unwired: 2 in, 1 out]
    n192 = Fract/Exp String To Number(use system decimal point (T)=FALSE, string=w350) -> (number=w84:dbl)  [unwired: 2 in, 1 out]
    n193 = Fract/Exp String To Number(use system decimal point (T)=FALSE, string=w330) -> (number=w82:dbl)  [unwired: 2 in, 1 out]
    n194 = Fract/Exp String To Number(use system decimal point (T)=FALSE, string=w332) -> (number=w80:dbl)  [unwired: 2 in, 1 out]
    n195 = Or(x="Clear_L3", y="Clear_L4") -> (x .or. y?=w127:bool)
    n196 = Multiply(x=w86, y=w82) -> (x*y=w81:dbl)
    "S2_I0" <- w81
    n197 = Multiply(x=w86, y=w80) -> (x*y=w79:dbl)
    "S2_I1" <- w79
    n198 = Multiply(x=w86, y=w78) -> (x*y=w77:dbl)
    "S2_I2" <- w77
    n199 = Multiply(x=w86, y=w76) -> (x*y=w75:dbl)
    "S2_I3" <- w75
    n200 = Multiply(x=w86, y=w83) -> (x*y=w74:dbl)
    "S2_I4" <- w74
    n201 = Multiply(x=w86, y=w84) -> (x*y=w85:dbl)
    "S2_I5" <- w85
    n202 = call "Read.vi"("R_Channel"="2", "R_Call_Function"=w511, "IP"="IP") -> ("R_Return"=w592:string)
    n203 = call "Read.vi"("R_Channel"="3", "R_Call_Function"=w511, "IP"="IP") -> ("R_Return"=w594:string)
    n204 = call "Read.vi"("R_Channel"="4", "R_Call_Function"=w511, "IP"="IP") -> ("R_Return"=w604:string)
    n205 = call "Read.vi"("R_Channel"="5", "R_Call_Function"=w511, "IP"="IP") -> ("R_Return"=w603:string)
    n206 = call "Read.vi"("R_Channel"="0", "R_Call_Function"=w511, "IP"="IP") -> ("R_Return"=w583:string)
    n207 = call "Read.vi"("R_Channel"="1", "R_Call_Function"=w511, "IP"="IP") -> ("R_Return"=w593:string)
    n208 = Match Pattern(string=w592, regular expression=" A") -> (before substring=w591:string)  [unwired: 1 in, 3 out]
    n209 = Match Pattern(string=w594, regular expression=" A") -> (before substring=w595:string)  [unwired: 1 in, 3 out]
    n210 = Match Pattern(string=w604, regular expression=" A") -> (before substring=w605:string)  [unwired: 1 in, 3 out]
    n211 = Match Pattern(string=w603, regular expression=" A") -> (before substring=w602:string)  [unwired: 1 in, 3 out]
    n212 = Match Pattern(string=w583, regular expression=" A") -> (before substring=w582:string)  [unwired: 1 in, 3 out]
    n213 = Match Pattern(string=w593, regular expression=" A") -> (before substring=w584:string)  [unwired: 1 in, 3 out]
    n214 = Build Array(w81, w79, w77, w75, w74, w85) -> (w272:dbl[])
    n215 = call "Channel plots.vi"("Current time"=w460, "In Channels"=w491, "Input Channels"=w272) -> ("output graph"=→"S2_1-6 Channels Current":T5, "out Ch 1"=w163:dbl[], "out Ch 6"=w153:dbl[], "out Ch 2"=w161:dbl[], "out Ch 3"=w159:dbl[], "out Ch 4"=w157:dbl[], "out Ch 5"=w155:dbl[])
    n216 = Fract/Exp String To Number(use system decimal point (T)=FALSE, string=w591) -> (number=w115:dbl)  [unwired: 2 in, 1 out]
    n217 = Fract/Exp String To Number(use system decimal point (T)=FALSE, string=w595) -> (number=w116:dbl)  [unwired: 2 in, 1 out]
    n218 = Fract/Exp String To Number(use system decimal point (T)=FALSE, string=w605) -> (number=w118:dbl)  [unwired: 2 in, 1 out]
    n219 = Fract/Exp String To Number(use system decimal point (T)=FALSE, string=w602) -> (number=w117:dbl)  [unwired: 2 in, 1 out]
    n220 = Fract/Exp String To Number(use system decimal point (T)=FALSE, string=w582) -> (number=w119:dbl)  [unwired: 2 in, 1 out]
    n221 = Fract/Exp String To Number(use system decimal point (T)=FALSE, string=w584) -> (number=w114:dbl)  [unwired: 2 in, 1 out]
    n222 = Multiply(x=w126, y=w119) -> (x*y=w113:dbl)
    "S1_I0" <- w113
    n223 = Multiply(x=w126, y=w114) -> (x*y=w112:dbl)
    "S1_I1" <- w112
    n224 = Multiply(x=w126, y=w115) -> (x*y=w111:dbl)
    "S1_I2" <- w111
    n225 = Multiply(x=w126, y=w116) -> (x*y=w110:dbl)
    "S1_I3" <- w110
    n226 = Multiply(x=w126, y=w118) -> (x*y=w109:dbl)
    "S1_I4" <- w109
    n227 = Multiply(x=w126, y=w117) -> (x*y=w108:dbl)
    "S1_I5" <- w108
    n228 = call "Read.vi"("R_Channel"="108", "R_Call_Function"=w283, "IP"=w282) -> ("R_Return"=w375:string)
    n229 = call "Read.vi"("R_Channel"="109", "R_Call_Function"=w283, "IP"=w282) -> ("R_Return"=w373:string)
    n230 = call "Read.vi"("R_Channel"="110", "R_Call_Function"=w283, "IP"=w282) -> ("R_Return"=w363:string)
    n231 = call "Read.vi"("R_Channel"="111", "R_Call_Function"=w283, "IP"=w282) -> ("R_Return"=w364:string)
    n232 = call "Read.vi"("R_Channel"="112", "R_Call_Function"=w283, "IP"=w282) -> ("R_Return"=w288:string)
    n233 = call "Read.vi"("R_Channel"="113", "R_Call_Function"=w283, "IP"=w282) -> ("R_Return"=w289:string)
    n234 = call "Read.vi"("R_Channel"="114", "R_Call_Function"=w283, "IP"=w282) -> ("R_Return"=w299:string)
    n235 = call "Read.vi"("R_Channel"="115", "R_Call_Function"=w283, "IP"=w282) -> ("R_Return"=w298:string)
    n236 = call "Read.vi"("R_Channel"="106", "R_Call_Function"=w283, "IP"=w282) -> ("R_Return"=w384:string)
    n237 = call "Read.vi"("R_Channel"="107", "R_Call_Function"=w283, "IP"=w282) -> ("R_Return"=w374:string)
    n238 = Match Pattern(string=w375, regular expression=" A") -> (before substring=w376:string)  [unwired: 1 in, 3 out]
    n239 = Match Pattern(string=w373, regular expression=" A") -> (before substring=w372:string)  [unwired: 1 in, 3 out]
    n240 = Match Pattern(string=w363, regular expression=" A") -> (before substring=w362:string)  [unwired: 1 in, 3 out]
    n241 = Match Pattern(string=w364, regular expression=" A") -> (before substring=w365:string)  [unwired: 1 in, 3 out]
    n242 = Match Pattern(string=w288, regular expression=" A") -> (before substring=w287:string)  [unwired: 1 in, 3 out]
    n243 = Match Pattern(string=w289, regular expression=" A") -> (before substring=w290:string)  [unwired: 1 in, 3 out]
    n244 = Match Pattern(string=w299, regular expression=" A") -> (before substring=w300:string)  [unwired: 1 in, 3 out]
    n245 = Match Pattern(string=w298, regular expression=" A") -> (before substring=w297:string)  [unwired: 1 in, 3 out]
    n246 = Build Array(w113, w112, w111, w110, w109, w108) -> (w277:dbl[])
    n247 = call "Channel plots.vi"("Current time"=w460, "In Channels"=w565, "Input Channels"=w277) -> ("output graph"=→"S1_1-6 Channels Current":T5, "out Ch 1"=w231:dbl[], "out Ch 6"=w221:dbl[], "out Ch 2"=w229:dbl[], "out Ch 3"=w227:dbl[], "out Ch 4"=w225:dbl[], "out Ch 5"=w223:dbl[])
    n248 = Match Pattern(string=w384, regular expression=" A") -> (before substring=w385:string)  [unwired: 1 in, 3 out]
    n249 = Match Pattern(string=w374, regular expression=" A") -> (before substring=w383:string)  [unwired: 1 in, 3 out]
    n250 = case shown="True" "stop" {
      tunnel: "stop" -> [_ w829]
      tunnel: [FALSE ("stop") w827] -> w264
      frame False {
      }
      frame True {
        n251 = flat-sequence {
          tunnel: w829 -> [w830]
          tunnel: [w830] -> w828
          tunnel: w828 -> [w832]
          tunnel: [w832] -> w826
          tunnel: w826 -> [w833]
          tunnel: [w833] -> w825
          tunnel: [w835] -> w827
          tunnel: w825 -> [w835]
          frame #0 {
            n252 = Wait (ms)(milliseconds to wait=u32 100) -> ()  [unwired: 1 out]
          }
          frame #1 {
          }
          frame #2 {
            n253 = Wait (ms)(milliseconds to wait=u32 100) -> ()  [unwired: 1 out]
          }
          frame #3 {
          }
        }
      }
    }
    n254 = Fract/Exp String To Number(use system decimal point (T)=FALSE, string=w376) -> (number=w70:dbl)  [unwired: 2 in, 1 out]
    n255 = Fract/Exp String To Number(use system decimal point (T)=FALSE, string=w372) -> (number=w69:dbl)  [unwired: 2 in, 1 out]
    n256 = Fract/Exp String To Number(use system decimal point (T)=FALSE, string=w362) -> (number=w68:dbl)  [unwired: 2 in, 1 out]
    n257 = Fract/Exp String To Number(use system decimal point (T)=FALSE, string=w365) -> (number=w67:dbl)  [unwired: 2 in, 1 out]
    n258 = Fract/Exp String To Number(use system decimal point (T)=FALSE, string=w287) -> (number=w66:dbl)  [unwired: 2 in, 1 out]
    n259 = Fract/Exp String To Number(use system decimal point (T)=FALSE, string=w290) -> (number=w65:dbl)  [unwired: 2 in, 1 out]
    n260 = Fract/Exp String To Number(use system decimal point (T)=FALSE, string=w300) -> (number=w64:dbl)  [unwired: 2 in, 1 out]
    n261 = Fract/Exp String To Number(use system decimal point (T)=FALSE, string=w297) -> (number=w63:dbl)  [unwired: 2 in, 1 out]
    n262 = Fract/Exp String To Number(use system decimal point (T)=FALSE, string=w385) -> (number=w72:dbl)  [unwired: 2 in, 1 out]
    n263 = Fract/Exp String To Number(use system decimal point (T)=FALSE, string=w383) -> (number=w71:dbl)  [unwired: 2 in, 1 out]
    n264 = Multiply(x=w73, y=w72) -> (x*y=w62:dbl)
    "S2_I6" <- w62
    n265 = Multiply(x=w73, y=w71) -> (x*y=w61:dbl)
    "S2_I7" <- w61
    n266 = Multiply(x=w73, y=w70) -> (x*y=w60:dbl)
    "S2_I8" <- w60
    n267 = Multiply(x=w73, y=w69) -> (x*y=w59:dbl)
    "S2_I9" <- w59
    n268 = Multiply(x=w73, y=w68) -> (x*y=w58:dbl)
    "S2_I10" <- w58
    n269 = Multiply(x=w73, y=w67) -> (x*y=w57:dbl)
    "S2_I11" <- w57
    n270 = Multiply(x=w73, y=w66) -> (x*y=w56:dbl)
    "S2_I12" <- w56
    n271 = Multiply(x=w73, y=w65) -> (x*y=w55:dbl)
    "S2_I13" <- w55
    n272 = Multiply(x=w73, y=w64) -> (x*y=w54:dbl)
    "S2_I14" <- w54
    n273 = Multiply(x=w73, y=w63) -> (x*y=w53:dbl)
    "S2_I15" <- w53
    n274 = call "Read.vi"("R_Channel"="8", "R_Call_Function"=w511, "IP"="IP") -> ("R_Return"=w627:string)
    n275 = call "Read.vi"("R_Channel"="9", "R_Call_Function"=w511, "IP"="IP") -> ("R_Return"=w625:string)
    n276 = call "Read.vi"("R_Channel"="10", "R_Call_Function"=w511, "IP"="IP") -> ("R_Return"=w615:string)
    n277 = call "Read.vi"("R_Channel"="11", "R_Call_Function"=w511, "IP"="IP") -> ("R_Return"=w616:string)
    n278 = call "Read.vi"("R_Channel"="12", "R_Call_Function"=w511, "IP"="IP") -> ("R_Return"=w517:string)
    n279 = call "Read.vi"("R_Channel"="13", "R_Call_Function"=w511, "IP"="IP") -> ("R_Return"=w518:string)
    n280 = call "Read.vi"("R_Channel"="14", "R_Call_Function"=w511, "IP"="IP") -> ("R_Return"=w528:string)
    n281 = call "Read.vi"("R_Channel"="15", "R_Call_Function"=w511, "IP"="IP") -> ("R_Return"=w527:string)
    n282 = call "Read.vi"("R_Channel"="6", "R_Call_Function"=w511, "IP"="IP") -> ("R_Return"=w636:string)
    n283 = call "Read.vi"("R_Channel"="7", "R_Call_Function"=w511, "IP"="IP") -> ("R_Return"=w626:string)
    n284 = Match Pattern(string=w627, regular expression=" A") -> (before substring=w628:string)  [unwired: 1 in, 3 out]
    n285 = Match Pattern(string=w625, regular expression=" A") -> (before substring=w624:string)  [unwired: 1 in, 3 out]
    n286 = Match Pattern(string=w615, regular expression=" A") -> (before substring=w614:string)  [unwired: 1 in, 3 out]
    n287 = Match Pattern(string=w616, regular expression=" A") -> (before substring=w617:string)  [unwired: 1 in, 3 out]
    n288 = Match Pattern(string=w517, regular expression=" A") -> (before substring=w516:string)  [unwired: 1 in, 3 out]
    n289 = Match Pattern(string=w518, regular expression=" A") -> (before substring=w519:string)  [unwired: 1 in, 3 out]
    n290 = Match Pattern(string=w528, regular expression=" A") -> (before substring=w529:string)  [unwired: 1 in, 3 out]
    n291 = Match Pattern(string=w527, regular expression=" A") -> (before substring=w526:string)  [unwired: 1 in, 3 out]
    n292 = Match Pattern(string=w636, regular expression=" A") -> (before substring=w637:string)  [unwired: 1 in, 3 out]
    n293 = Match Pattern(string=w626, regular expression=" A") -> (before substring=w635:string)  [unwired: 1 in, 3 out]
    n294 = Build Array(w56, w55, w54, w53) -> (w270:dbl[])
    n295 = call "Channel plots.vi"("Current time"=w460, "In Channels"=w503, "Input Channels"=w270) -> ("output graph"=→"S2_13-16 Channels Current":T5, "out Ch 1"=w139:dbl[], "out Ch 2"=w137:dbl[], "out Ch 3"=w135:dbl[], "out Ch 4"=w133:dbl[])  [unwired: 2 out]
    n296 = Build Array(w62, w61, w60, w59, w58, w57) -> (w271:dbl[])
    n297 = call "Channel plots.vi"("Current time"=w460, "In Channels"=w478, "Input Channels"=w271) -> ("output graph"=→"S2_6-12 Channels Current":T5, "out Ch 1"=w151:dbl[], "out Ch 6"=w141:dbl[], "out Ch 2"=w149:dbl[], "out Ch 3"=w147:dbl[], "out Ch 4"=w145:dbl[], "out Ch 5"=w143:dbl[])
    n298 = case shown="False" w127 {
      tunnel: w195 -> [w777 _]
      tunnel: [w777 w778] -> w194
      tunnel: [w776 w778] -> w192
      tunnel: w193 -> [w776 _]
      tunnel: [w775 w778] -> w190
      tunnel: w191 -> [w775 _]
      tunnel: w189 -> [w774 _]
      tunnel: [w774 w778] -> w188
      tunnel: [w773 w778] -> w186
      tunnel: w187 -> [w773 _]
      tunnel: [w772 w778] -> w184
      tunnel: w185 -> [w772 _]
      tunnel: w183 -> [w771 _]
      tunnel: [w771 w778] -> w182
      tunnel: w181 -> [w770 _]
      tunnel: [w770 w778] -> w180
      tunnel: w179 -> [w769 _]
      tunnel: [w769 w778] -> w178
      tunnel: [w768 w778] -> w176
      tunnel: w177 -> [w768 _]
      tunnel: w175 -> [w767 _]
      tunnel: [w767 w778] -> w174
      tunnel: [w766 w778] -> w172
      tunnel: w173 -> [w766 _]
      tunnel: w171 -> [w765 _]
      tunnel: [w765 w778] -> w170
      tunnel: [w764 w778] -> w168
      tunnel: w169 -> [w764 _]
      tunnel: w167 -> [w763 _]
      tunnel: [w763 w778] -> w166
      tunnel: w165 -> [w762 _]
      tunnel: [w762 w778] -> w164
      tunnel: w163 -> [w761 _]
      tunnel: [w761 w778] -> w162
      tunnel: w161 -> [w760 _]
      tunnel: [w760 w778] -> w160
      tunnel: w159 -> [w759 _]
      tunnel: [w759 w778] -> w158
      tunnel: w157 -> [w758 _]
      tunnel: [w758 w778] -> w156
      tunnel: w155 -> [w757 _]
      tunnel: [w757 w778] -> w154
      tunnel: w153 -> [w756 _]
      tunnel: [w756 w778] -> w152
      tunnel: w151 -> [w755 _]
      tunnel: [w755 w778] -> w150
      tunnel: w149 -> [w754 _]
      tunnel: [w754 w778] -> w148
      tunnel: w147 -> [w753 _]
      tunnel: [w753 w778] -> w146
      tunnel: w145 -> [w752 _]
      tunnel: [w752 w778] -> w144
      tunnel: w143 -> [w751 _]
      tunnel: [w751 w778] -> w142
      tunnel: w141 -> [w750 _]
      tunnel: [w750 w778] -> w140
      tunnel: [w749 w778] -> w138
      tunnel: w139 -> [w749 _]
      tunnel: w137 -> [w748 _]
      tunnel: [w748 w778] -> w136
      tunnel: w135 -> [w747 _]
      tunnel: [w747 w778] -> w134
      tunnel: w133 -> [w746 _]
      tunnel: [w746 w778] -> w132
      tunnel: w130 -> [_ w778]
      frame False {
      }
      frame True {
      }
    }
    n299 = Fract/Exp String To Number(use system decimal point (T)=FALSE, string=w628) -> (number=w105:dbl)  [unwired: 2 in, 1 out]
    n300 = Fract/Exp String To Number(use system decimal point (T)=FALSE, string=w624) -> (number=w104:dbl)  [unwired: 2 in, 1 out]
    n301 = Fract/Exp String To Number(use system decimal point (T)=FALSE, string=w614) -> (number=w103:dbl)  [unwired: 2 in, 1 out]
    n302 = Fract/Exp String To Number(use system decimal point (T)=FALSE, string=w617) -> (number=w102:dbl)  [unwired: 2 in, 1 out]
    n303 = Fract/Exp String To Number(use system decimal point (T)=FALSE, string=w516) -> (number=w94:dbl)  [unwired: 2 in, 1 out]
    n304 = Fract/Exp String To Number(use system decimal point (T)=FALSE, string=w519) -> (number=w89:dbl)  [unwired: 2 in, 1 out]
    n305 = Fract/Exp String To Number(use system decimal point (T)=FALSE, string=w529) -> (number=w88:dbl)  [unwired: 2 in, 1 out]
    n306 = Fract/Exp String To Number(use system decimal point (T)=FALSE, string=w526) -> (number=w87:dbl)  [unwired: 2 in, 1 out]
    n307 = Fract/Exp String To Number(use system decimal point (T)=FALSE, string=w637) -> (number=w107:dbl)  [unwired: 2 in, 1 out]
    n308 = Fract/Exp String To Number(use system decimal point (T)=FALSE, string=w635) -> (number=w106:dbl)  [unwired: 2 in, 1 out]
    n309 = Build Array (concatenate)(w272, w271, w270) -> (→"S2_Current":dbl[])
    n310 = Multiply(x=w93, y=w107) -> (x*y=w101:dbl)
    "S1_I6" <- w101
    n311 = Multiply(x=w93, y=w106) -> (x*y=w100:dbl)
    "S1_I7" <- w100
    n312 = Multiply(x=w93, y=w105) -> (x*y=w99:dbl)
    "S1_I8" <- w99
    n313 = Multiply(x=w93, y=w104) -> (x*y=w98:dbl)
    "S1_I9" <- w98
    n314 = Multiply(x=w93, y=w103) -> (x*y=w97:dbl)
    "S1_I10" <- w97
    n315 = Multiply(x=w93, y=w102) -> (x*y=w96:dbl)
    "S1_I11" <- w96
    n316 = Multiply(x=w93, y=w94) -> (x*y=w90:dbl)
    "S1_I12" <- w90
    n317 = Multiply(x=w93, y=w89) -> (x*y=w95:dbl)
    "S1_I13" <- w95
    n318 = Multiply(x=w93, y=w88) -> (x*y=w91:dbl)
    "S1_I14" <- w91
    n319 = Multiply(x=w93, y=w87) -> (x*y=w92:dbl)
    "S1_I15" <- w92
    n320 = Build Array(w90, w95, w91, w92) -> (w275:dbl[])
    n321 = call "Channel plots.vi"("Current time"=w460, "In Channels"=w506, "Input Channels"=w275) -> ("output graph"=→"S1_13-16 Channels Current":T5, "out Ch 1"=w207:dbl[], "out Ch 2"=w205:dbl[], "out Ch 3"=w203:dbl[], "out Ch 4"=w201:dbl[])  [unwired: 2 out]
    n322 = Build Array(w101, w100, w99, w98, w97, w96) -> (w276:dbl[])
    n323 = call "Channel plots.vi"("Current time"=w460, "In Channels"=w578, "Input Channels"=w276) -> ("output graph"=→"S1_6-12 Channels Current":T5, "out Ch 1"=w219:dbl[], "out Ch 6"=w209:dbl[], "out Ch 2"=w217:dbl[], "out Ch 3"=w215:dbl[], "out Ch 4"=w213:dbl[], "out Ch 5"=w211:dbl[])
    n324 = Build Array (concatenate)(w277, w276, w275) -> (→"S1_Current":dbl[])
    n325 = case shown="False" w197 {
      tunnel: w263 -> [w822 _]
      tunnel: [w822 w823] -> w262
      tunnel: [w821 w823] -> w261
      tunnel: w260 -> [w821 _]
      tunnel: [w820 w823] -> w258
      tunnel: w259 -> [w820 _]
      tunnel: w257 -> [w819 _]
      tunnel: [w819 w823] -> w256
      tunnel: [w818 w823] -> w254
      tunnel: w255 -> [w818 _]
      tunnel: [w817 w823] -> w253
      tunnel: w252 -> [w817 _]
      tunnel: w251 -> [w816 _]
      tunnel: [w816 w823] -> w250
      tunnel: w249 -> [w815 _]
      tunnel: [w815 w823] -> w248
      tunnel: w247 -> [w814 _]
      tunnel: [w814 w823] -> w246
      tunnel: [w813 w823] -> w244
      tunnel: w245 -> [w813 _]
      tunnel: w243 -> [w812 _]
      tunnel: [w812 w823] -> w242
      tunnel: [w811 w823] -> w240
      tunnel: w241 -> [w811 _]
      tunnel: w239 -> [w810 _]
      tunnel: [w810 w823] -> w238
      tunnel: [w809 w823] -> w236
      tunnel: w237 -> [w809 _]
      tunnel: w235 -> [w808 _]
      tunnel: [w808 w823] -> w234
      tunnel: w233 -> [w807 _]
      tunnel: [w807 w823] -> w232
      tunnel: w231 -> [w806 _]
      tunnel: [w806 w823] -> w230
      tunnel: w229 -> [w805 _]
      tunnel: [w805 w823] -> w228
      tunnel: w227 -> [w804 _]
      tunnel: [w804 w823] -> w226
      tunnel: w225 -> [w803 _]
      tunnel: [w803 w823] -> w224
      tunnel: w223 -> [w802 _]
      tunnel: [w802 w823] -> w222
      tunnel: w221 -> [w801 _]
      tunnel: [w801 w823] -> w220
      tunnel: w219 -> [w800 _]
      tunnel: [w800 w823] -> w218
      tunnel: w217 -> [w799 _]
      tunnel: [w799 w823] -> w216
      tunnel: w215 -> [w798 _]
      tunnel: [w798 w823] -> w214
      tunnel: w213 -> [w797 _]
      tunnel: [w797 w823] -> w212
      tunnel: w211 -> [w796 _]
      tunnel: [w796 w823] -> w210
      tunnel: w209 -> [w795 _]
      tunnel: [w795 w823] -> w208
      tunnel: [w794 w823] -> w206
      tunnel: w207 -> [w794 _]
      tunnel: w205 -> [w793 _]
      tunnel: [w793 w823] -> w204
      tunnel: w203 -> [w792 _]
      tunnel: [w792 w823] -> w202
      tunnel: w201 -> [w791 _]
      tunnel: [w791 w823] -> w200
      tunnel: w130 -> [_ w823]
      frame False {
      }
      frame True {
      }
    }
    "Numeric" <- w45
  }
